vi "Format Log.vi"(7 "Timestamps":bool, 8 "error in (no error)":errorcluster, 10 "Items":T1[](array[typedef]) {"Time" format="%<%H:%M:%S>T"}, 11 "LV Chat Server in":refnum<class "LV Chat Server.lvclass">) -> (0 "error out":errorcluster, 2 "Log":string, 3 "LV Chat Server out":refnum<class "LV Chat Server.lvclass">)   [LabVIEW 2020, in "LV Chat Server.lvclass"]
uses:
  LV Chat Server.lvclass
  Data Types/Message.ctl
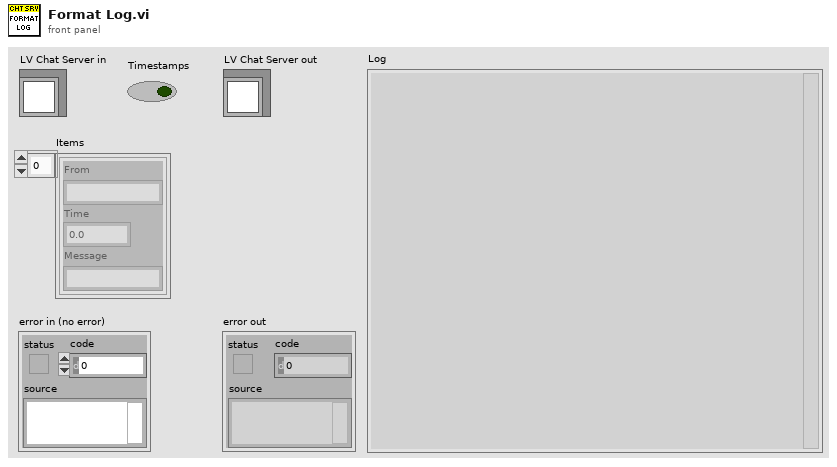
[diagram p1: front panel]
types:
  T1 = typedef "Message.ctl" = cluster{"From":string, "Time":dbl, "Message":string}
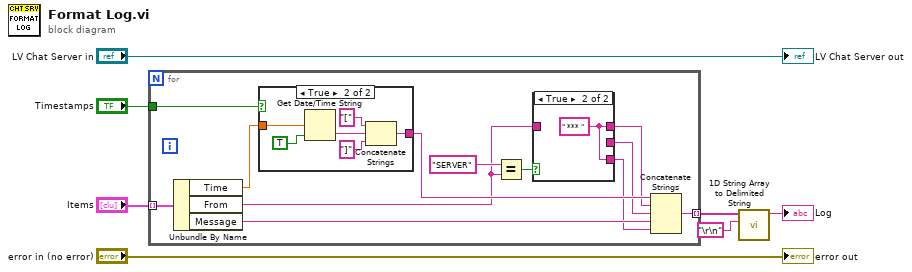
[diagram p0: block diagram]
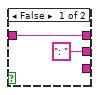
[diagram p2: hidden frame]
diagram:
  n1 = for {
    tunnel: "Items" -> [w19] mode=indexing
    tunnel: "Timestamps" -> [w18]
    tunnel: [w14] -> w3 mode=indexing
    n2 = Unbundle By Name(w19) -> ("Time"=w17:dbl, "From"=w11:string, "Message"=w16:string)
    n3 = case shown="True" w18 {
      tunnel: w17 -> [_ w28]
      tunnel: [_ w23] -> w15
      frame False {
      }
      frame True {
        n4 = Get Date/Time String(seconds (now)=w28, want seconds? (F)=TRUE) -> (time string=w26:string)  [unwired: 1 in, 1 out]
        n5 = Concatenate Strings("[" ("string"), w26, "]" ("string")) -> (w23:string)
      }
    }
    n6 = Equal?(x="SERVER", y=w11) -> (x = y?=w12:bool)
    n7 = case shown="True" w12 {
      tunnel: w11 -> [w21 _]
      tunnel: [w21 w22] -> w10
      tunnel: [": " ("string") _] -> w9
      tunnel: [_ w22] -> w8
      frame False {
      }
      frame True {
        w22 = " *** " ("From")
      }
    }
    n8 = Concatenate Strings(w15, w10, w9, w16, w8) -> (w14:string)
  }
  n9 = call <vilib>:"1D String Array to Delimited String.vi"("delimiter"="\r\n", "string array"=w3) -> ("delimited string"=→"Log":string)  [unwired: 9 in]
  "error out" <- "error in (no error)"
  "LV Chat Server out" <- "LV Chat Server in"
